vi "Find And Replace One VI.vi"(8 "error in (no error)":errorcluster, 10 "VI Ref in":refnum<vi>, 11 "MetaDataObj":refnum<class "MetaDataObj.lvclass">) -> (0 "error out":errorcluster, 2 "VI Ref out":refnum<vi>)   [LabVIEW 2016, in "MetaDataObj.lvclass"]
uses:
  <resource>/dialog/NewProjectWizard/MetaDataObj/MetaDataObj.lvclass
  <vilib>/Utility/traverseref.llb/TRef TravTarget.ctl
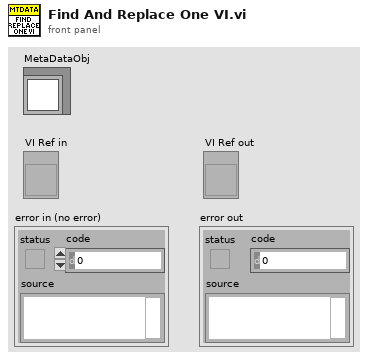
[diagram p1: front panel]
types:
  T1 = enum32{"invalid VI type", "Standard VI", "Control VI", "Global VI", "Polymorphic VI", "Configuration VI", "SubSystem", "Facade VI", "Method VI", "Statechart Diagram VI"}
  T2 = typedef "TRef TravTarget.ctl" = enum16{"FP", "BD", "Other"}
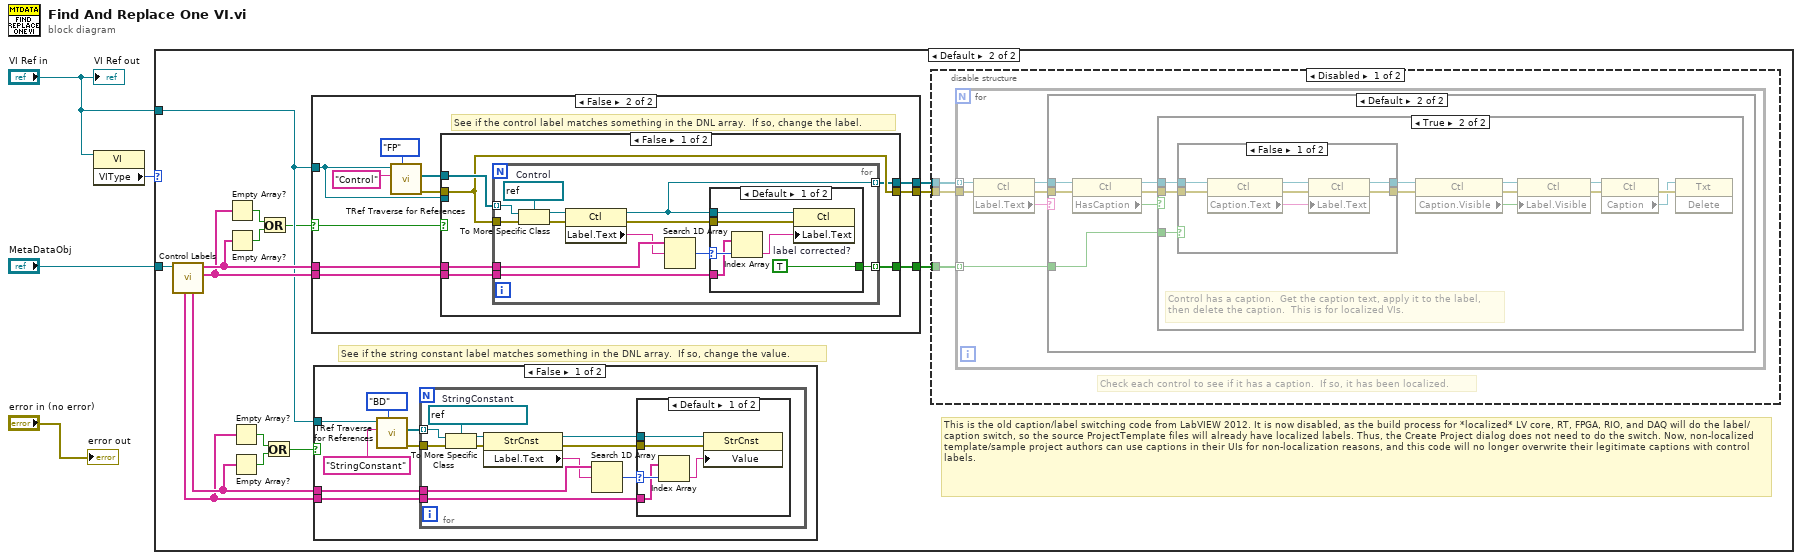
[diagram p0: block diagram]
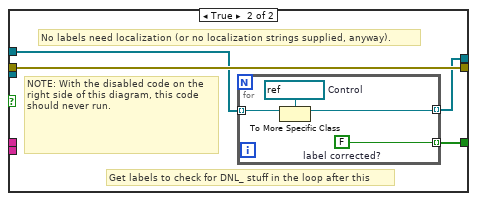
[diagram p5: hidden frame]
diagram:
  n1 = property class="VI"(reference="VI Ref in") -> ("VIType"=w1:T1)  [unwired: 1 in, 2 out]
  n2 = case shown="Default" w1 {
    tunnel: "MetaDataObj" -> [_ w17]
    tunnel: "VI Ref in" -> [_ w6]
    frame "Global VI" {
      # "Do not alter controls on global VIs with localized content because changing the label of a control in a global breaks the callers."
    }
    frame Default {
      # "This is the old caption/label switching code from LabVIEW 2012. It is now disabled, as the build process for *localized* LV core, RT, FPGA, RIO, and DAQ will do the label/caption switch, so the source ProjectTemplate files will already have localized labels. Thus, the Create Project dialog does not need to do the switch. Now, non-localized template/sample project authors can use captions in their UIs for non-localization reasons, and this code will no longer overwrite their legitimate captions with control labels."
      # "See if the string constant label matches something in the DNL array.  If so, change the value."
      n3 = call-dynamic "Control Labels.vi"("MetaDataObj.lvclass"=w17) -> ("localized control labels"=w15:string[], "DNL_unlocalized control labels"=w16:string[], "DNL_unlocalized string constant labels"=w11:string[], "localized string constant values"=w10:string[])  [unwired: 7 in]
      n4 = Empty Array?(array=w15) -> (empty?=w19:bool)
      n5 = Empty Array?(array=w16) -> (empty?=w18:bool)
      n6 = Empty Array?(array=w10) -> (empty?=w12:bool)
      n7 = Empty Array?(array=w11) -> (empty?=w13:bool)
      n8 = Or(x=w19, y=w18) -> (x .or. y?=w5:bool)
      n9 = Or(x=w12, y=w13) -> (x .or. y?=w14:bool)
      n10 = case shown="False" w5 {
        selector: w5 -> [_ w20]
        tunnel: w16 -> [_ w30]
        tunnel: w15 -> [_ w29]
        tunnel: [_ w25] -> w9
        tunnel: [_ w23] -> w8
        tunnel: [_ w22] -> w7
        tunnel: w6 -> [_ w21]
        frame True {
          # "No special localized control labels specified for this template/sample project"
        }
        frame False {
          # "See if the control label matches something in the DNL array.  If so, change the label."
          n11 = call <vilib>:"TRef Traverse for References.vi"("Traverse Target"=TRef_TravTarget."FP", "Class Name"="Control", "VI Refnum"=w21) -> ("error out"=w26:errorcluster, "References"=w24:refnum<vi>[])  [unwired: 2 in, 5 out]
          n12 = case shown="False" w20 {
            tunnel: w21 -> [_ _]
            tunnel: w30 -> [w36 _]
            tunnel: w29 -> [w35 _]
            tunnel: w24 -> [w34 w57]
            tunnel: w26 -> [w33 w58]
            tunnel: [w33 w58] -> w25
            tunnel: [w32 w56] -> w23
            tunnel: [w31 w55] -> w22
            frame False {
              n13 = for {
                tunnel: w34 -> [w46] mode=indexing
                tunnel: w33 -> [w44]
                tunnel: w36 -> [w42]
                tunnel: w35 -> [w40]
                tunnel: [w38] -> w32 mode=indexing
                tunnel: [w37] -> w31 mode=indexing
                w47 = refnum<vi> refnum  # Control
                n14 = To More Specific Class(target class=w47, reference=w46, error in=w44) -> (specific class reference=w45:refnum<vi>, error out=w43:errorcluster)
                n15 = property class="Ctl"(reference=w45, error in=w43) -> (reference out=w38:refnum<vi>, error out=w48:errorcluster, "Label.Text"=w39:string)
                n16 = Search 1D Array(1D array=w42, element=w39) -> (index of element=w41:i32)  [unwired: 1 in]
                n17 = case shown="Default" w41 {
                  selector: w41 -> [w52 _]
                  tunnel: w38 -> [w54 _]
                  tunnel: w48 -> [w53 _]
                  tunnel: w40 -> [w51 _]
                  tunnel: [w49 _] -> w37
                  frame Default {
                    w49 = TRUE  # label corrected?
                    n18 = Index Array(array=w51, index=w52) -> (element=w50:string)
                    n19 = property class="Ctl"(reference=w54, error in=w53, "Label.Text"=w50) -> ()  [unwired: 2 out]
                  }
                  frame -1 {
                  }
                }
              }
            }
            frame True {
              # "NOTE: With the disabled code on the right side of this diagram, this code should never run."
              # "Get labels to check for DNL_ stuff in the loop after this"
              # "No labels need localization (or no localization strings supplied, anyway)."
              n20 = for {
                tunnel: [w60] -> w56 mode=indexing
                tunnel: w57 -> [w61] mode=indexing
                tunnel: [w59] -> w55 mode=indexing
                w59 = FALSE  # label corrected?
                w62 = refnum<vi> refnum  # Control
                n21 = To More Specific Class(target class=w62, reference=w61) -> (specific class reference=w60:refnum<vi>)  [unwired: 1 in, 1 out]
              }
            }
          }
        }
      }
      n22 = case shown="False" w14 {
        tunnel: w6 -> [w101 _]
        tunnel: w11 -> [w105 _]
        tunnel: w10 -> [w104 _]
        frame False {
          n23 = call <vilib>:"TRef Traverse for References.vi"("Traverse Target"=TRef_TravTarget."BD", "Class Name"="StringConstant", "VI Refnum"=w101) -> ("error out"=w99:errorcluster, "References"=w100:refnum<vi>[])  [unwired: 2 in, 5 out]
          n24 = for {
            tunnel: w100 -> [w113] mode=indexing
            tunnel: w99 -> [w111]
            tunnel: w105 -> [w109]
            tunnel: w104 -> [w106]
            w114 = refnum<vi> refnum  # StringConstant
            n25 = To More Specific Class(target class=w114, reference=w113, error in=w111) -> (specific class reference=w112:refnum<vi>, error out=w110:errorcluster)
            n26 = property class="StrCnst"(reference=w112, error in=w110) -> (reference out=w116:refnum<vi>, error out=w115:errorcluster, "Label.Text"=w108:string)
            n27 = Search 1D Array(1D array=w109, element=w108) -> (index of element=w107:i32)  [unwired: 1 in]
            n28 = case shown="Default" w107 {
              selector: w107 -> [w119 _]
              tunnel: w116 -> [w121 _]
              tunnel: w115 -> [w120 _]
              tunnel: w106 -> [w118 _]
              frame Default {
                n29 = Index Array(array=w118, index=w119) -> (element=w117:string)
                n30 = property class="StrCnst"(reference=w121, error in=w120, "Value"=w117) -> ()  [unwired: 2 out]
              }
              frame -1 {
              }
            }
          }
        }
        frame True {
          # "No string constants need localization (or no localization strings supplied, anyway)."
        }
      }
      n31 = disable-structure shown="Disabled" {
        disable-tunnel: w9 -> [w65 _]
        disable-tunnel: w8 -> [w64 _]
        disable-tunnel: w7 -> [w63 _]
        frame Disabled {
          # "Check each control to see if it has a caption.  If so, it has been localized."
          n32 = for {
            tunnel: w65 -> [w71]
            tunnel: w64 -> [w68] mode=indexing
            tunnel: w63 -> [w70] mode=indexing
            n33 = property class="Ctl"(reference=w68, error in=w71) -> (reference out=w67:refnum<vi>, error out=w69:errorcluster, "Label.Text"=w66:string)
            n34 = case shown="Default" w66 {
              tunnel: w70 -> [_ w74]
              tunnel: w69 -> [_ w73]
              tunnel: w67 -> [_ w72]
              frame "error in", "error in (no error)", "error out" {
                # "Do not do the caption/label switch on error clusters."
              }
              frame Default {
                n35 = property class="Ctl"(reference=w72, error in=w73) -> (reference out=w75:refnum<vi>, error out=w76:errorcluster, "HasCaption"=w77:bool)
                n36 = case shown="True" w77 {
                  tunnel: w76 -> [_ w89]
                  tunnel: w75 -> [_ w88]
                  tunnel: w74 -> [_ w85]
                  frame False {
                    # "Ignore controls without captions"
                  }
                  frame True {
                    # "Control has a caption.  Get the caption text, apply it to the label,\nthen delete the caption.  This is for localized VIs."
                    n37 = case shown="False" w85 {
                      tunnel: w89 -> [w96 w97]
                      tunnel: w88 -> [w95 w98]
                      tunnel: [w91 w98] -> w79
                      tunnel: [w90 w97] -> w82
                      frame False {
                        n38 = property class="Ctl"(reference=w95, error in=w96) -> (reference out=w94:refnum<vi>, error out=w93:errorcluster, "Caption.Text"=w92:string)
                        n39 = property class="Ctl"(reference=w94, error in=w93, "Label.Text"=w92) -> (reference out=w91:refnum<vi>, error out=w90:errorcluster)
                      }
                      frame True {
                        # "Label.Text was already corrected"
                      }
                    }
                    n40 = property class="Ctl"(reference=w79, error in=w82) -> (reference out=w81:refnum<vi>, error out=w80:errorcluster, "Caption.Visible"=w78:bool)
                    n41 = property class="Ctl"(reference=w81, error in=w80, "Label.Visible"=w78) -> (reference out=w83:refnum<vi>, error out=w84:errorcluster)
                    n42 = property class="Ctl"(reference=w83, error in=w84) -> (error out=w87:errorcluster, "Caption"=w86:refnum<vi>)  [unwired: 1 out]
                    n43 = invoke class="Txt" method="Delete"(reference=w86, error in=w87) -> ()  [unwired: 1 in, 3 out]
                  }
                }
              }
            }
          }
        }
        frame Enabled {
        }
      }
    }
  }
  "error out" <- "error in (no error)"
  "VI Ref out" <- "VI Ref in"
